vi "Error_log.vi"(11 "error in (no error)":errorcluster) -> (2 "Error Log":string[][](table), 15 "error out":errorcluster)   [LabVIEW 2023, in "task_1.lvlib"]
doc: "Use dto catch the error event and log it onto the table"
uses:
  task_1.lvlib
  Controls/event_operations.ctl
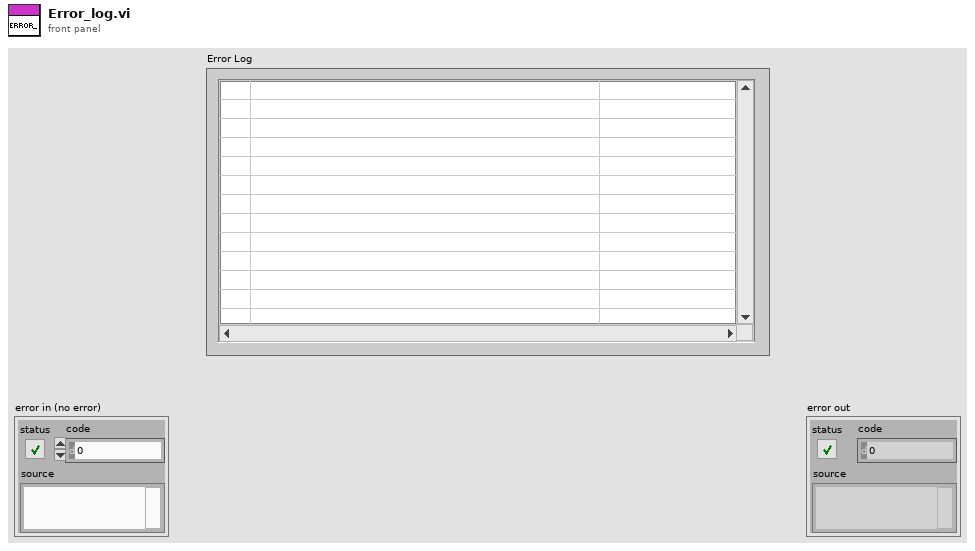
[diagram p1: front panel]
types:
  T1 = typedef "task_1.lvlib/event_operations.ctl" = enum16{"Create", "Generate", "Destroy"}
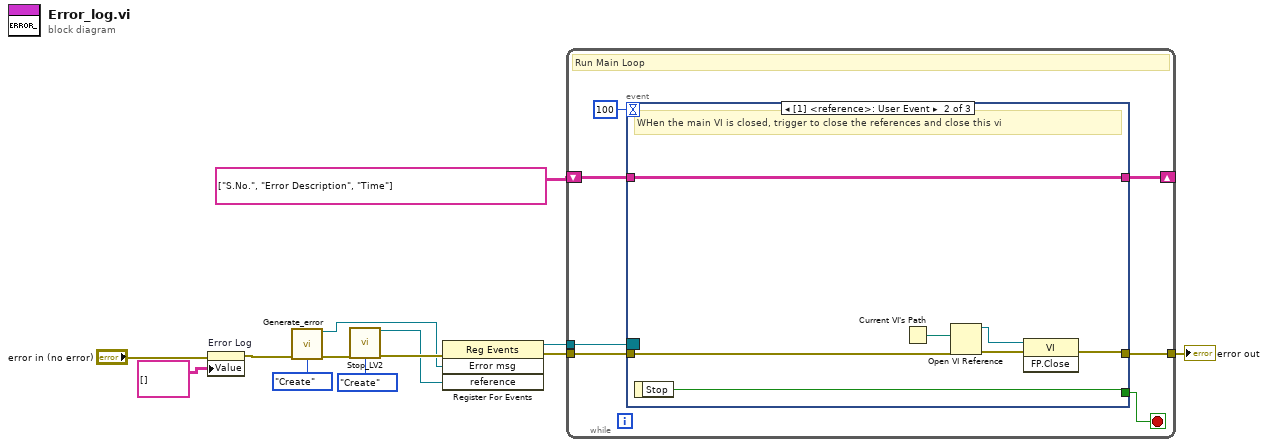
[diagram p0: block diagram]
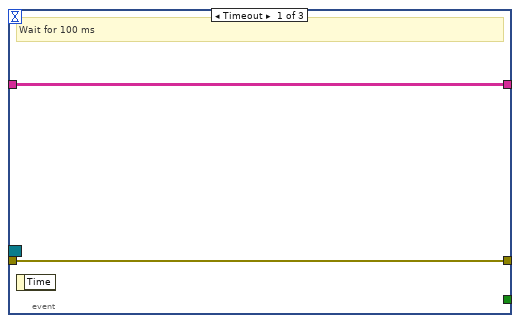
[diagram p2: hidden frame]
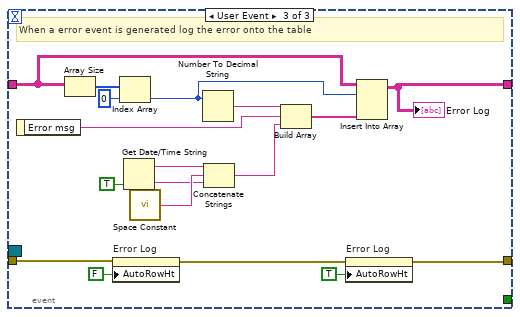
[diagram p3: hidden frame]
diagram:
  n1 = property on="Error Log" class="Tbl (strict)"(error in="error in (no error)", "Value"=string[][] [] ("Error Log")) -> (error out=w4:errorcluster)  [unwired: 1 in, 1 out]
  n2 = call "Generate_error.vi"("error in (no error)"=w4, "Operations"=event_operations."Create") -> ("Error msg"=w2:refnum<user-event>, "error IO"=w3:errorcluster)  [unwired: 12 in]
  n3 = call "Stop_LV2.vi"("error in (no error)"=w3, "Operations"=event_operations."Create") -> ("reference"=w8:refnum<user-event>, "error out"=w10:errorcluster)  [unwired: 12 in]
  n4 = register-events(error in=w10, w2, w8) -> (reference out=w12:refnum<event-registration>, error out=w13:errorcluster)  [unwired: 1 in]
  n5 = while {
    tunnel: w13 -> [w20]
    tunnel: [w19] -> w7
    tunnel: w12 -> [w18]
    shift-right: [w15] -> _
    shift-left: string[][] [["S.No.", "Error Description", "Time"]] -> [w16]
    stop <- w14 stop-if-true
    # "Run Main Loop"
    n6 = event shown="[1] <reference>: User Event" {
      selector: w18 -> [_ _ _]
      dyn-events: _ -> [_ _ _]
      timeout: 100 -> [_ _ _]
      tunnel: w20 -> [w22 w29 w36]
      tunnel: [w22 w25 w32] -> w19
      tunnel: w16 -> [w21 w28 w40]
      tunnel: [w21 w28 w38] -> w15
      tunnel: [_ w23 _] -> w14
      event Timeout {
        # "Wait for 100 ms"
        n7 = event-data() -> ()  [unwired: 1 in, 1 out]
      }
      event User Event {
        # "WHen the main VI is closed, trigger to close the references and close this vi"
        n8 = event-data() -> ("Stop"=w23:bool)  [unwired: 1 in]
        n9 = Current VI's Path() -> (path=w26:path)
        n10 = Open VI Reference(vi path=w26, error in (no error)=w29) -> (vi reference=w24:refnum<vi>, error out=w27:errorcluster)  [unwired: 4 in]
        n11 = invoke class="VI" method="FP.Close"(reference=w24, error in=w27) -> (error out=w25:errorcluster)  [unwired: 1 in, 2 out]
      }
      event User Event {
        # "When a error event is generated log the error onto the table"
        n12 = event-data() -> ("Error msg"=w44:string)  [unwired: 1 in]
        n13 = Array Size(array=w40) -> (size(s)=w47:i32[])
        n14 = property on="Error Log" class="Tbl (strict)"(error in=w36, "AutoRowHt"=FALSE ("Autosizing Row Height")) -> (error out=w33:errorcluster)  [unwired: 1 in, 1 out]
        n15 = Index Array(array=w47, index=0) -> (element=w37:i32)
        n16 = Get Date/Time String(want seconds? (F)=TRUE) -> (date string=w42:string, time string=w30:string)  [unwired: 2 in]
        n17 = call <vilib>:"Space Constant.vi"() -> ("String"=w31:string)
        n18 = Number To Decimal String(number=w37) -> (decimal integer string=w45:string)  [unwired: 1 in]
        n19 = Concatenate Strings(w42, w31, w30) -> (w41:string)
        n20 = Build Array(w45, w44, w41) -> (w39:string[])
        n21 = property on="Error Log" class="Tbl (strict)"(error in=w33, "AutoRowHt"=TRUE ("Autosizing Row Height")) -> (error out=w32:errorcluster)  [unwired: 1 in, 1 out]
        n22 = Insert Into Array(array=w40, index (row)=w37, new element=w39) -> (w38:string[][])  [unwired: 1 in]
        "Error Log" <- w38
      }
    }
  }
  "error out" <- w7
